vi "Generate signal pulses.vi"() -> ()   [LabVIEW 2010]
doc: "This example shows how to generate signal pulses of predefined signal waveforms like sine, triangle, square, ramp up, ramp down or pwm). Generated signal can be observed by Red Pitaya Oscilloscope WEB application. To run it, just open web browser, input Red Pitaya IP and start Oscilloscope. On Oscilloscope set acquisition mode to Single, Trigger to 100mV and time range relative to frequency of a signal."
uses:
  RedPitaya.lvlib
panel:
  in  "Trigger Source":u16(ring)=5 items=["", "EXT_PE", "EXT_NE", "INT", "GATED", "IMM", "IMM BOTH"]
  in  "Total Time of One Burst":i32=-1
  in  "Number of repeated Bursts":string
  in  "Number of generated Signals / Burst":string="1"
  in  "Frequency":i32=10
  in  "Amplitude":dbl=1.0
  in  "Waveform Function":u16(ring)=1 items=["", "Sine", "Square", "Triangle", "Sawtooth UP", "Sawtooth Down", "PWM"]
  in  "Channel (1|2)":u16(ring)=1 items=["Channel 1"=1, "Channel 2"=2]
  in  "IP address":string="192.168.1.100"
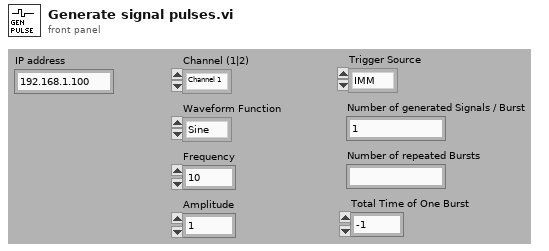
[diagram p1: front panel]
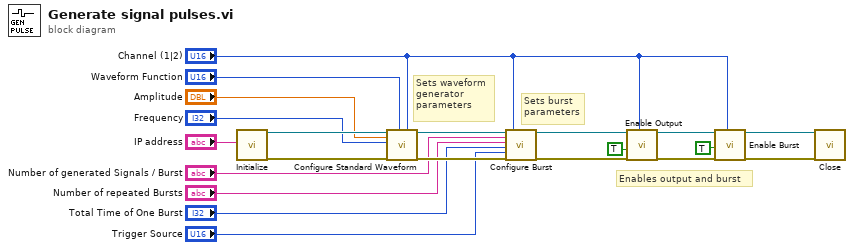
[diagram p0: block diagram]
diagram:
  # "Enables output and burst"
  # "Sets burst\nparameters"
  # "Sets waveform\ngenerator\nparameters"
  n1 = call "Initialize.vi"("IP address"="IP address") -> ("RedPitaya TCP Connection"=w19:refnum<k5>, "error out"=w18:errorcluster)  [unwired: 17 in]
  n2 = call "Configure Standard Waveform.vi"("RedPitaya connection in"=w19, "Amplitude"="Amplitude", "Frequency"="Frequency", "error in"=w18, "Channel #"="Channel (1|2)", "Waveform Function"="Waveform Function") -> ("RedPitaya connection out"=w17:refnum<k5>, "error out"=w15:errorcluster)  [unwired: 12 in]
  n3 = call "Configure Burst.vi"("RedPitaya connection in"=w17, "Number of generated Signals / Burst"="Number of generated Signals / Burst", "Number of repeated Bursts"="Number of repeated Bursts", "Total time of One Burst"="Total Time of One Burst", "Trigger Source"="Trigger Source", "error in"=w15, "Channel #"="Channel (1|2)") -> ("RedPitaya connection out"=w16:refnum<k5>, "error out"=w14:errorcluster)  [unwired: 11 in]
  n4 = call "Enable Output.vi"("RedPitaya connection in"=w16, "Generation (T: Enable)"=TRUE, "error in"=w14, "Channel #"="Channel (1|2)") -> ("RedPitaya connection out"=w13:refnum<k5>, "error out"=w12:errorcluster)  [unwired: 14 in]
  n5 = call "Enable Burst.vi"("RedPitaya connection in"=w13, "Generation (T: Enable)"=TRUE, "error in"=w12, "Channel #"="Channel (1|2)") -> ("RedPitaya connection out"=w10:refnum<k5>, "error out"=w9:errorcluster)  [unwired: 14 in]
  n6 = call "Close.vi"("connection ID"=w10, "error in"=w9) -> ()  [unwired: 17 in, 1 out]
